vi "Build Description String.vi"(8 "error in (no error)":errorcluster, 11 "Action Step in":refnum<class "Action Step.lvclass">) -> (0 "error out":errorcluster, 2 "Description":string, 3 "Action Step out":refnum<class "Action Step.lvclass">)   [LabVIEW 2020, in "MacroAssert.lvlib" / "Action Step.lvclass"]
doc: "Builds a string to describe what <B>Step</B> does."
uses:
  Action Step.lvclass
  C:/Users/User/Documents/LabVIEW Data/Projects/MacroAssert/source/Classes/Step/Step.lvclass
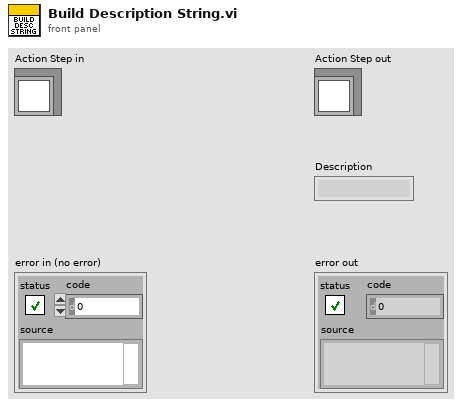
[diagram p1: front panel]
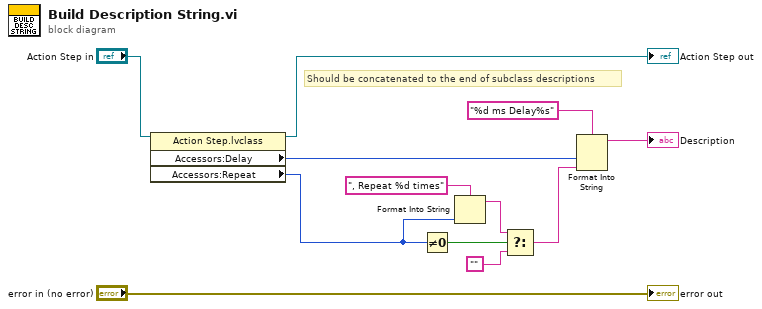
[diagram p0: block diagram]
diagram:
  # "Should be concatenated to the end of subclass descriptions"
  n1 = property class="Action Step.lvclass"(reference="Action Step in") -> (reference out=→"Action Step out":refnum<class "Action Step.lvclass">, "Accessors:Delay"=w3:i32, "Accessors:Repeat"=w4:i32)  [unwired: 1 in, 1 out]
  n2 = Not Equal To 0?(x=w4) -> (x != 0?=w11:bool)
  n3 = Format Into String(format string=", Repeat %d times", w4) -> (resulting string=w10:string)  [unwired: 2 in, 1 out]
  n4 = Select(t=w10, s=w11, f="") -> (s? t:f=w2:string)
  n5 = Format Into String(format string="%d ms Delay%s", w3, w2) -> (resulting string=→"Description":string)  [unwired: 2 in, 1 out]
  "error out" <- "error in (no error)"
